vi "CheckWhetherStartupOpState.vi"(8 "Error In":errorcluster, 11 "map in":T1) -> (0 "Error Out":errorcluster, 2 "Statrup Opstate?":bool, 3 "map out":T1)   [LabVIEW 2017, in "McsaDataEventCreator.lvlib"]
uses:
  <vilib>/addons/InsightCM/Devices/Shared/Mcsa/McsaDataEventCreator/McsaDataEventCreator.lvlib
  <vilib>/addons/PointValueMap/controls/PointMap.ctl
  <vilib>/addons/PointValueMap/subVIs/Point_Read_string.vi
  <vilib>/addons/PointValueMap/PointValueMap.lvlib
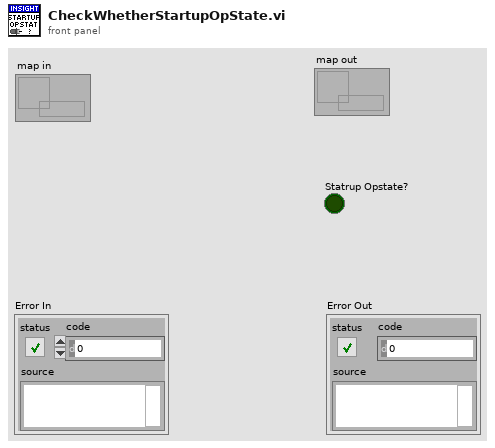
[diagram p1: front panel]
types:
  T1 = typedef "PointValueMap.lvlib/PointMap.ctl" = refnum<data-value>
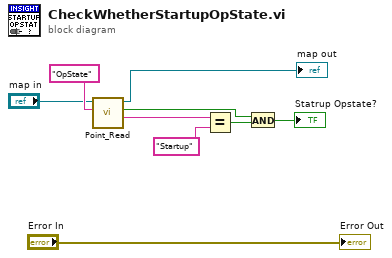
[diagram p0: block diagram]
diagram:
  n1 = call-poly <vilib>:"Point_Read.vi"("Tag"="OpState", "Map"="map in") -> ("Value"=w8:string, "Found?"=w5:bool, "Map Out"=→"map out":T1)  [unwired: 4 in, 3 out]
  n2 = Equal?(x=w8, y="Startup") -> (x = y?=w6:bool)
  n3 = And(x=w5, y=w6) -> (x .and. y?=→"Statrup Opstate?":bool)
  "Error Out" <- "Error In"
